vi "Process.vi"(8 "error in":errorcluster, 11 "Transport":refnum<class "Transport.lvclass">) -> (0 "error out":errorcluster, 3 "Transport out":refnum<class "Transport.lvclass">)   [LabVIEW 2016, in "Transport.lvclass"]
doc: "---------------------------------------------------------------\nJKI State Machine Objects™\nhttp://jki.net/state-machine-objects/\nCopyright (C) 2005-2015, JKI <info@jki.net>\nALL RIGHTS RESERVED"
uses:
  Transport.lvclass
  <vilib>/JKI/JKI SMO/SMO/SMO.lvclass
  <vilib>/JKI/JKI SMO/SMO/Typedefs/Parent Call--Enum.ctl
  Control Experiment/Control Experiment.lvclass
  <userlib>/LevyLab/Lockin-Multichannel/Instrument.Lockin/Instrument.Lockin.lvclass
  <userlib>/LevyLab/Levylab Instruments/Instrument Types/Cryostat/Typedefs/Magnet Axis--Enum.ctl
  <userlib>/LevyLab/Levylab Instruments/Instrument Types/Cryostat/Instrument.Cryostat.lvclass
  <userlib>/LevyLab/Levylab Instruments/Instrument Types/Cryostat/Typedefs/Magnet Mode--Enum.ctl
  <userlib>/LevyLab/Levylab Instruments/Instrument Types/Strain/Instrument.Strain.lvclass
  <userlib>/LevyLab/Levylab Instruments/Instrument Types/Optical Delay Line/Instrument.OpticalDelayLine.lvclass
  <userlib>/LevyLab/Levylab Instruments/Instrument Types/CBridge/Instrument.CBridge.lvclass
  C:/Program Files (x86)/National Instruments/LabVIEW 2016/vi.lib/JKI/JKI SMO/SMO/SMO.lvclass
panel:
  # "For instructions on how to use the JKI State Machine Objects, examples and video tutorials, visit:\nhttp://jki.net/state-machine-objects/\n\nJKI State Machine Objects™\nhttp://jki.net/state-machine-objects/\nCopyright (C) 2005-2015, JKI <info@jki.net>\nALL RIGHTS RESERVED"
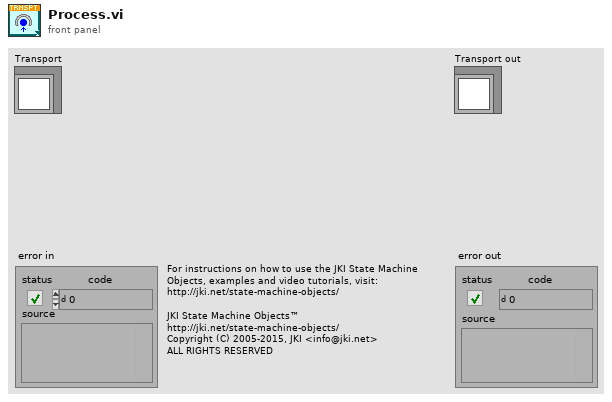
[diagram p1: front panel]
types:
  T1 = typedef "SMO.lvclass/Parent Call--Enum.ctl" = enum16{"Allows parent to run", "Does not request parent to run"}
  T2 = enum32{"invalid app kind", "Development System", "Run Time System", "Student Edition", "Embedded LabVIEW", "Evaluation", "Custom"}
  T3 = enum32{"Invalid", "Standard", "Closed", "Hidden", "Minimized", "Maximized"}
  T4 = enum32{"Bad", "Idle", "Run top level", "Running"}
  T5 = typedef "Instrument.Cryostat.lvclass/Magnet Mode--Enum.ctl" = enum16{"Persistent", "Driven"}
  T6 = typedef "Instrument.Cryostat.lvclass/Magnet Axis--Enum.ctl" = enum16{"Z", "X", "Y"}
  T7 = typedef "Control Experiment.lvclass/Instruments--cluster.ctl" = cluster{"Lockin":refnum<class "Instrument.Lockin.lvclass">, "Temperature":refnum<class "Instrument.Cryostat.lvclass">, "Magnet":refnum<class "Instrument.Cryostat.lvclass">, "Rotator":refnum<class "Instrument.Cryostat.lvclass">, "Level":refnum<class "Instrument.Cryostat.lvclass">, "C Bridge":refnum<class "Instrument.CBridge.lvclass">, "Optical Delay Line":refnum<class "Instrument.OpticalDelayLine.lvclass">, "Strain Cell":refnum<class "Instrument.Strain.lvclass">, "VNA":refnum<class "Instrument.VNA.lvclass">, "Voltage Source":refnum<class "Instrument.VSource.lvclass">, "KH7008":refnum<class "Instrument.KH7008.lvclass">[]}
  T8 = cluster{"Core":cluster{"Current VI Reference":refnum<vi>, "Close Panel on Exit?":bool, "error":errorcluster}, "Self Reference":refnum<class "Transport.lvclass">, "Control Experiment":refnum<class "Control Experiment.lvclass">, "Instruments":T7, "value":variant, "wait":bool}
  T9 = cluster{"Current VI Reference":refnum<vi>, "Close Panel on Exit?":bool, "error":errorcluster}
  T10 = typedef "SMO.lvclass/Protected Events.ctl" = cluster{"StopProcesses":refnum<user-event>, "AbortProcesses":refnum<user-event>, "Config Changed":refnum<user-event>, "Dependency":refnum<user-event>}
  T11 = typedef "Transport.lvclass/PrivateEvents--Cluster.ctl" = cluster{"Configure":refnum<user-event>}
  T12 = typedef "Lockin.DAQ.lvclass/State-enum.ctl" = enum16{"idle", "created", "started", "stopped", "sweeping"}
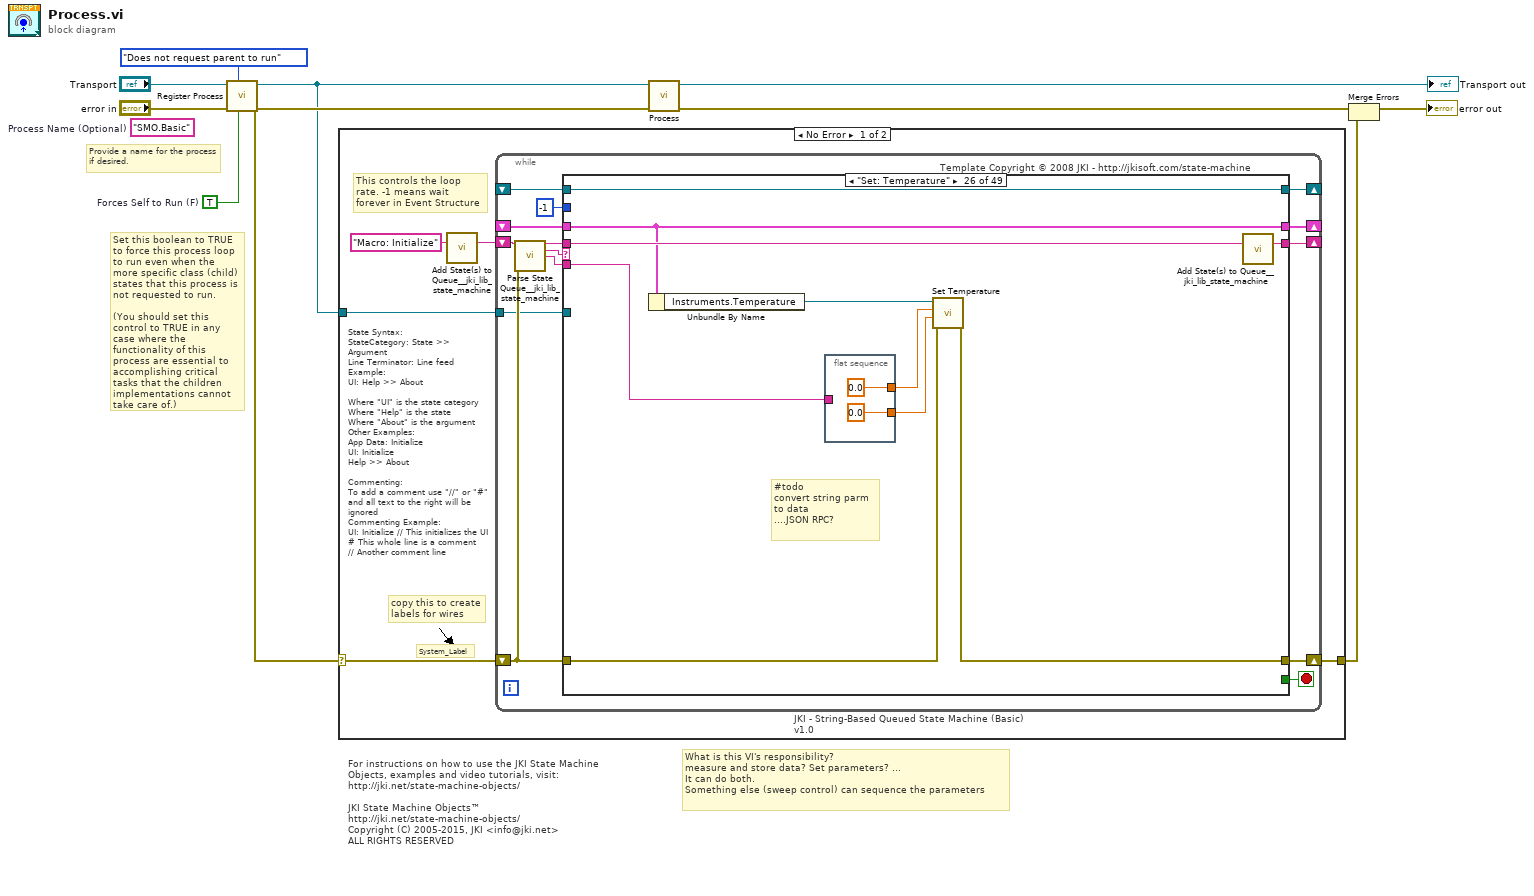
[diagram p0: block diagram]
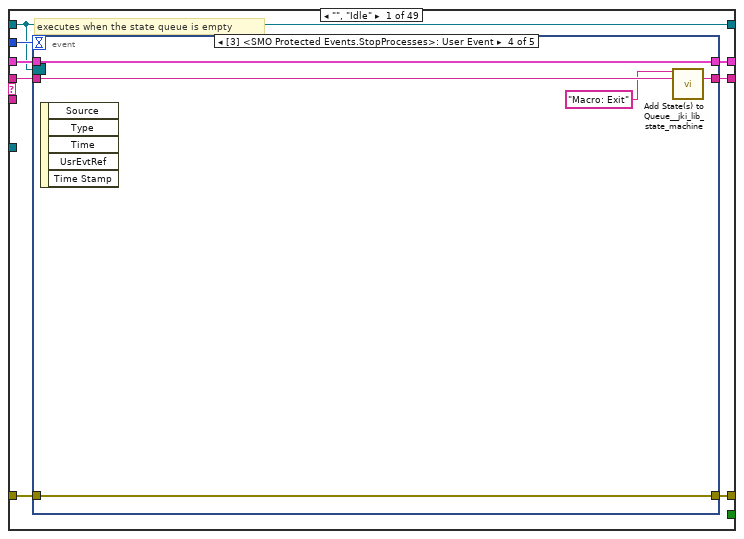
[diagram p2: hidden frame]
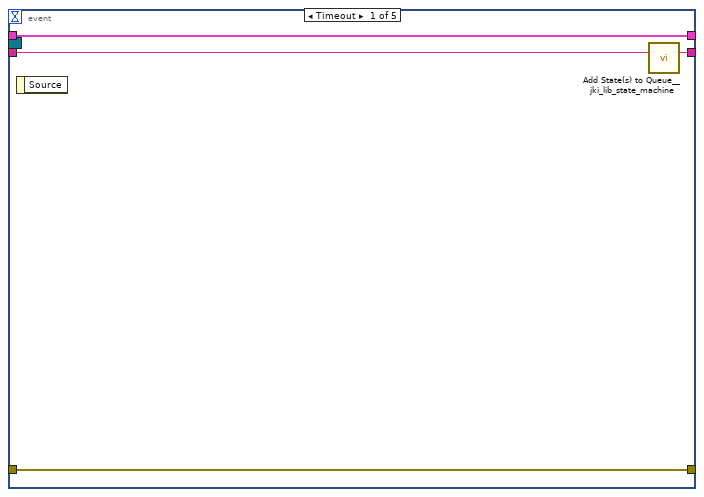
[diagram p3: hidden frame]
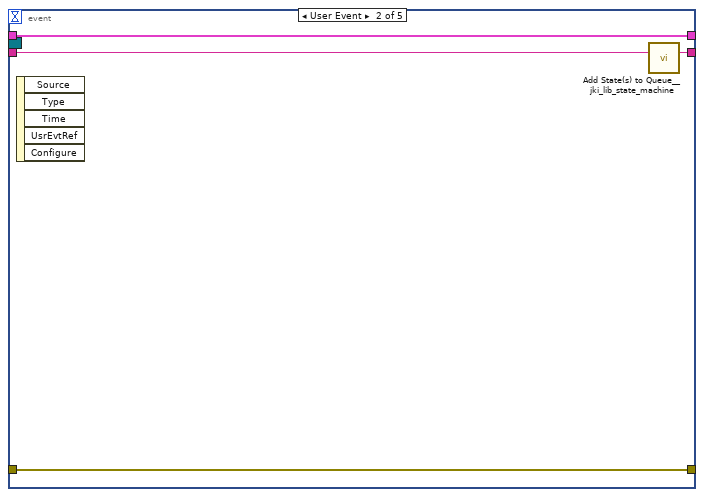
[diagram p4: hidden frame]
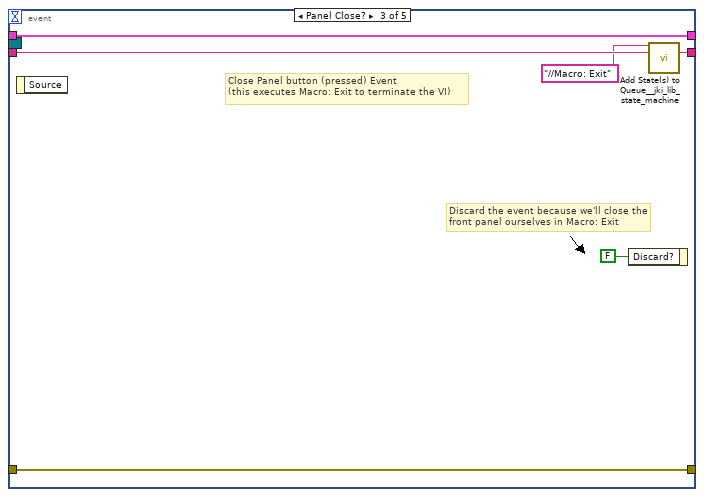
[diagram p5: hidden frame]
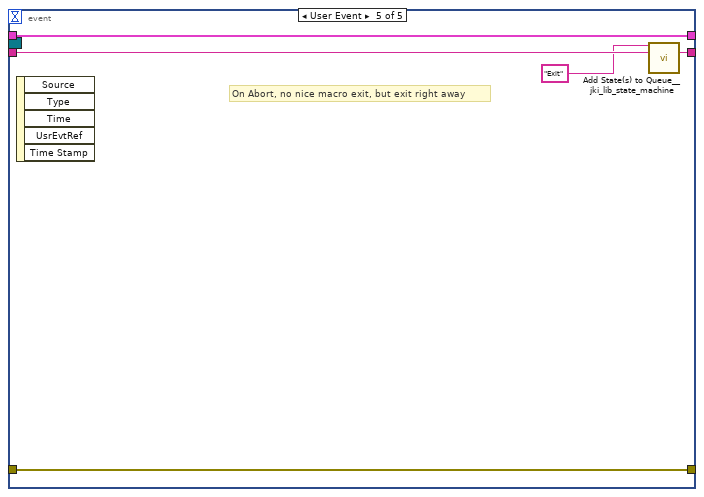
[diagram p6: hidden frame]
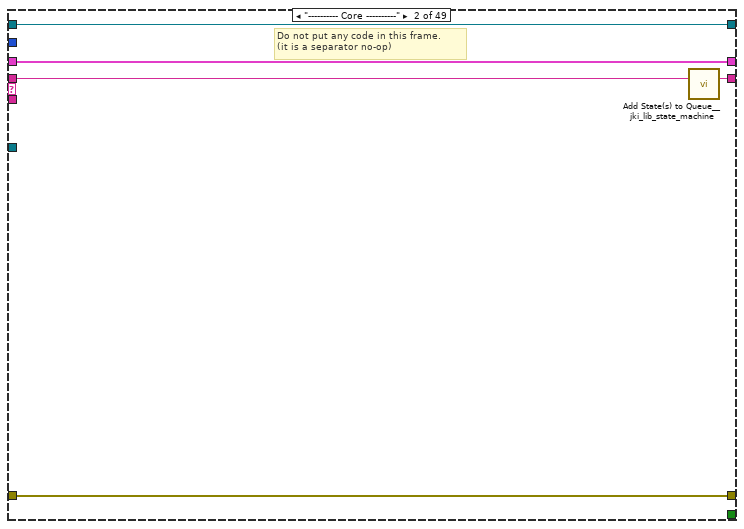
[diagram p7: hidden frame]
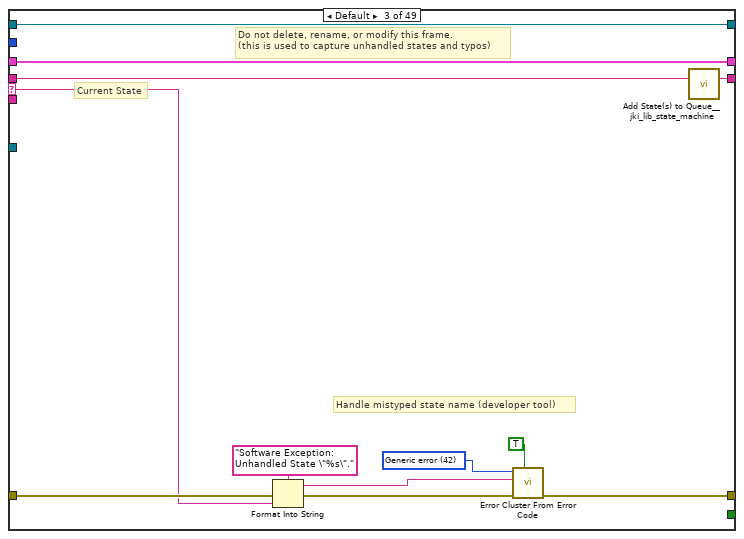
[diagram p8: hidden frame]
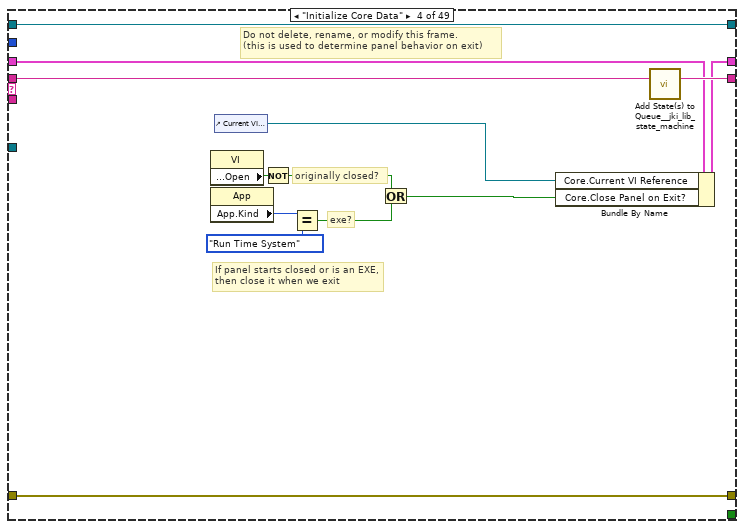
[diagram p9: hidden frame]
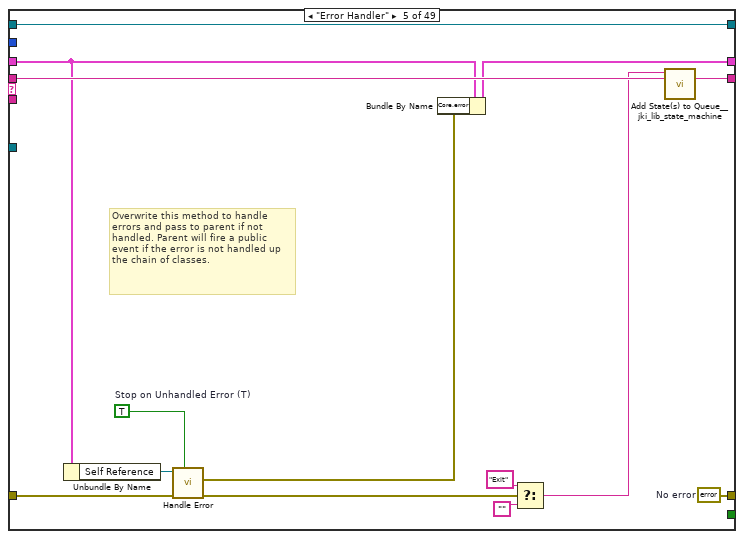
[diagram p10: hidden frame]
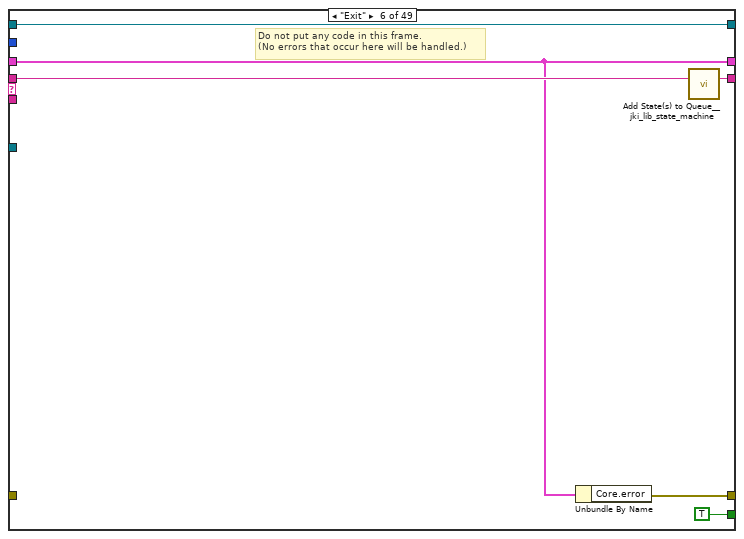
[diagram p11: hidden frame]
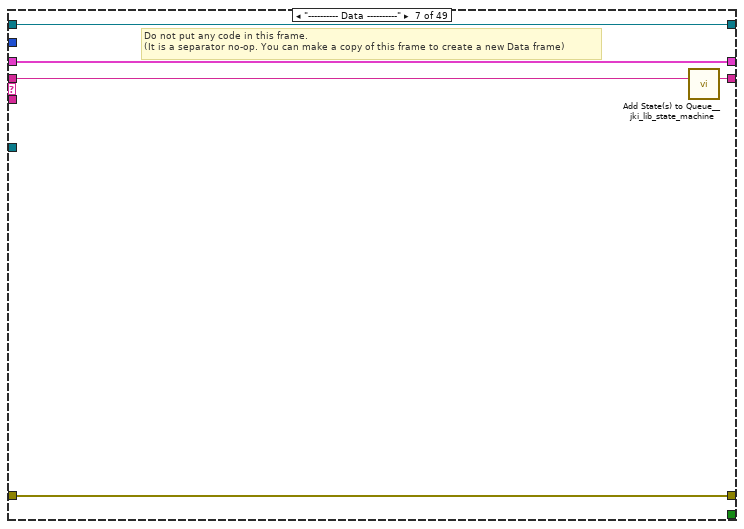
[diagram p12: hidden frame]
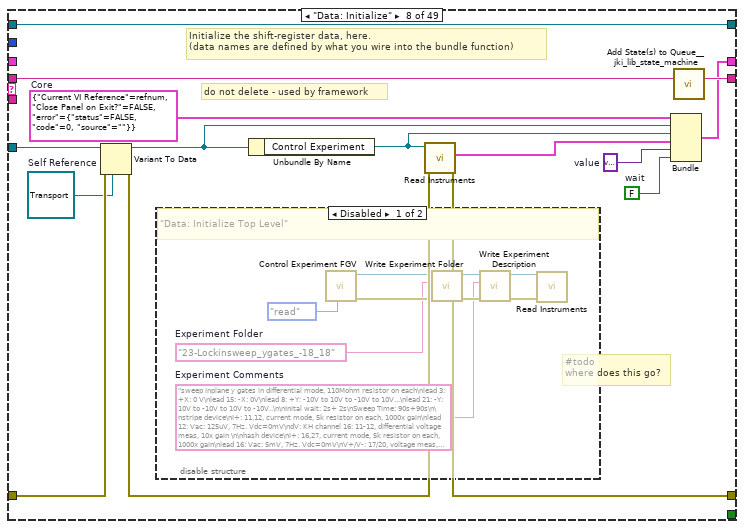
[diagram p13: hidden frame]
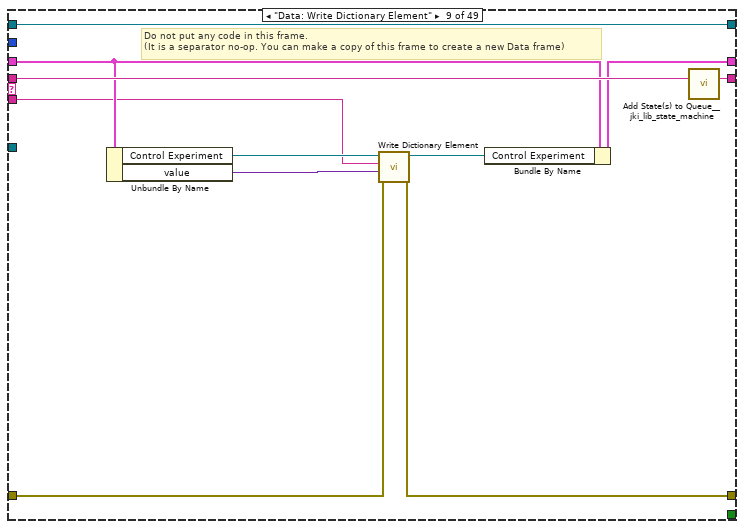
[diagram p15: hidden frame]
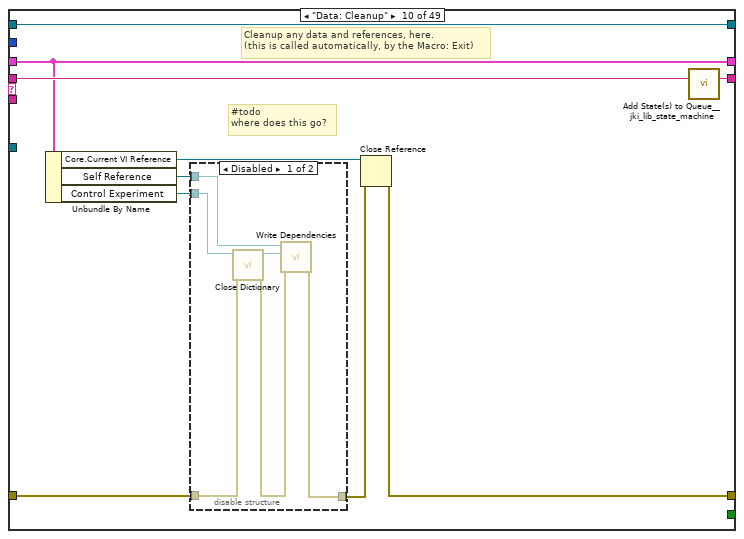
[diagram p16: hidden frame]
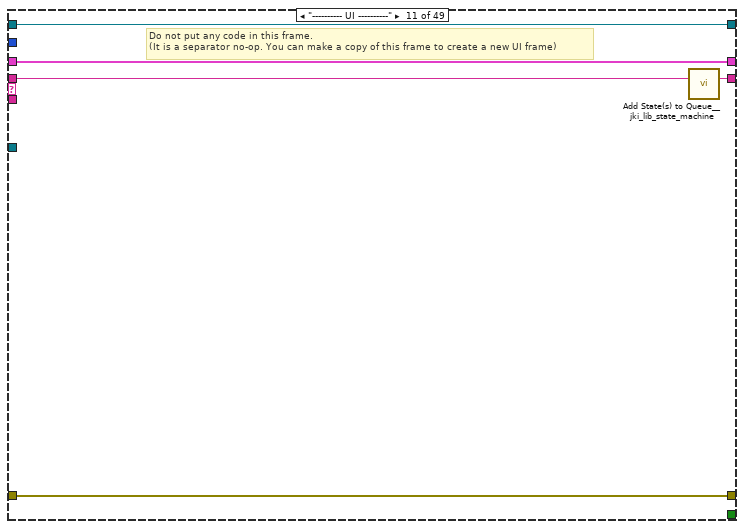
[diagram p18: hidden frame]
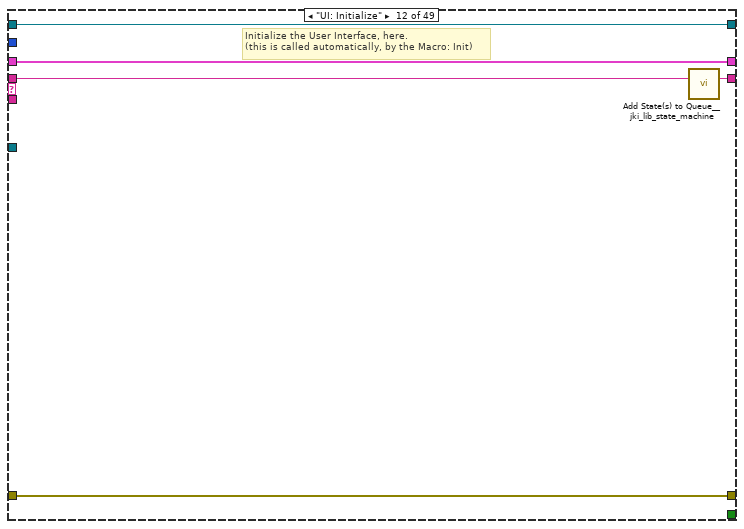
[diagram p19: hidden frame]
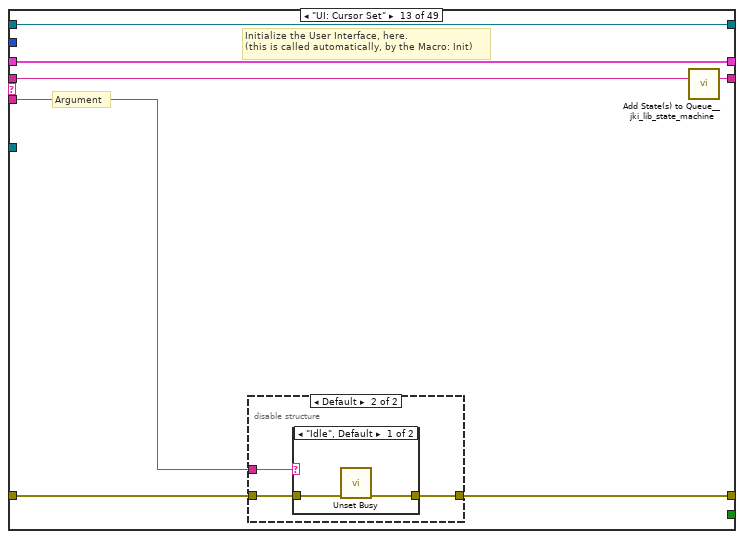
[diagram p20: hidden frame]
diagram:
  w1 = TRUE  # Forces Self to Run (F)
  (unwired) "SMO.Basic"  # Process Name (Optional)
  # "What is this VI's responsibility?\nmeasure and store data? Set parameters? ...\nIt can do both.\nSomething else (sweep control) can sequence the parameters"
  # "Provide a name for the process\nif desired."
  # "Set this boolean to TRUE to force this process loop to run even when the more specific class (child) states that this process is not requested to run.\n\n(You should set this control to TRUE in any case where the functionality of this process are essential to accomplishing critical tasks that the children implementations cannot take care of.)"
  # "For instructions on how to use the JKI State Machine Objects, examples and video tutorials, visit:\nhttp://jki.net/state-machine-objects/\n\nJKI State Machine Objects™\nhttp://jki.net/state-machine-objects/\nCopyright (C) 2005-2015, JKI <info@jki.net>\nALL RIGHTS RESERVED"
  n1 = call <vilib>:"Register Process.vi"("Forces Self to Run (F)"=w1, "Parent Call"=Parent_Call--Enum."Does not request parent to run", "error in (no error)"="error in", "SMO"="Transport") -> ("error out"=w7:errorcluster, "SMO out"=w6:refnum<class "Transport.lvclass">)  [unwired: 6 in]
  n2 = case shown="No Error" w7 {
    selector: w7 -> [w12 w561]
    tunnel: w6 -> [w13 _]
    tunnel: [w11 w561] -> w3
    frame No Error {
      # "State Syntax:\nStateCategory: State >> Argument\nLine Terminator: Line feed\nExample:\nUI: Help >> About\n\nWhere \"UI\" is the state category\nWhere \"Help\" is the state\nWhere \"About\" is the argument\nOther Examples:\nApp Data: Initialize\nUI: Initialize\nHelp >> About\n\nCommenting:\nTo add a comment use \"//\" or \"#\" and all text to the right will be ignored\nCommenting Example:\nUI: Initialize // This initializes the UI\n# This whole line is a comment\n// Another comment line"
      # "copy this to create labels for wires"
      # "This controls the loop rate. -1 means wait forever in Event Structure"
      # "System_Label"
      n3 = call <vilib>:"Add State(s) to Queue__jki_lib_state_machine.vi"("State(s) in (\"\")"="Macro: Initialize") -> ("States Out"=w15:string)  [unwired: 14 in]
      n4 = while "JKI - String-Based Queued State Machine (Basic) v1.0" {
        shift-right: [w22] -> _
        shift-left: _ -> [w21]
        shift-right: [w25] -> w11
        shift-left: w12 -> [w19]
        shift-right: [w24] -> _
        shift-left: w15 -> [w26]
        tunnel: w13 -> [w18]
        shift-right: [w17] -> _
        shift-left: _ -> [w16]
        stop <- w23 stop-if-true
        # "Template Copyright © 2008 JKI - http://jkisoft.com/state-machine"
        n5 = call <vilib>:"Parse State Queue__jki_lib_state_machine.vi"("State Queue"=w26, "Error In (no error)"=w19) -> ("Remaining States"=w28:string, "Current State"=w29:string, "Arguments"=w27:string)  [unwired: 11 in]
        n6 = case shown="\"Set: Temperature\"" w29 {
          selector: w29 -> [_ _ w68 _ _ _ _ _ _ _ _ _ _ _ _ _ _ _ _ _ _ _ _ _ w313 _ _ _ _ _ _ _ _ _ _ _ _ _ _ _ _ _ _ _ _ _ _ _ _]
          tunnel: w28 -> [w37 w66 w72 w91 w105 w111 w116 w131 w151 w161 w173 w178 w185 w201 w233 w247 w252 w266 w271 w282 w287 w299 w305 w310 w325 w335 w349 w363 w375 w387 w399 w411 w423 w435 w442 w449 w458 w467 w475 w480 w488 w497 w506 w515 w524 w533 w542 w551 w560]
          tunnel: w27 -> [_ _ _ _ _ _ _ _ w141 _ _ _ w179 w195 _ _ _ _ _ _ _ _ _ _ w314 w326 w344 w358 w370 w382 w394 w406 w418 w430 _ _ _ _ _ _ _ _ _ _ _ _ _ _ _]
          tunnel: w21 -> [w35 w63 w70 w82 w99 w107 w113 _ w146 w152 w170 w176 w183 w197 w230 w243 w249 w257 w268 w279 w284 w297 w303 w307 w321 w331 w345 w359 w371 w383 w395 w407 w419 w431 w439 w446 w455 w464 w472 w478 w485 w491 w500 w509 w518 w527 w536 w545 w554]
          tunnel: [w34 w64 w74 w88 w100 w106 w114 w119 w143 w158 w171 w175 w180 w198 w231 w245 w250 w264 w269 w273 w285 w293 w301 w308 w323 w332 w346 w360 w372 w384 w396 w408 w420 w432 w440 w443 w450 w459 w469 w476 w482 w493 w502 w511 w520 w529 w538 w547 w556] -> w25
          tunnel: w19 -> [w33 w64 w73 w88 w101 _ w114 w128 w144 w154 w171 w175 w181 w199 w231 w245 w250 w264 w269 w274 w285 w294 w301 w308 w323 w327 w338 w354 w366 w378 w390 w402 w414 w426 w440 w444 w453 w462 w470 w476 w482 w489 w498 w507 w516 w525 w534 w543 w552]
          tunnel: [w36 w65 w71 w90 w104 w110 w115 w130 w150 w160 w172 w177 w184 w200 w232 w246 w251 w265 w270 w281 w286 w298 w304 w309 w324 w334 w348 w362 w374 w386 w398 w410 w422 w434 w441 w448 w457 w466 w474 w479 w487 w496 w505 w514 w523 w532 w541 w550 w559] -> w24
          tunnel: [_ _ _ _ _ TRUE _ _ _ _ _ _ _ _ _ _ _ _ _ _ _ _ _ _ _ _ _ _ _ _ _ _ _ _ _ _ _ _ _ _ _ _ _ _ _ _ _ _ _] -> w23
          tunnel: [w32 w63 w70 w89 w98 w107 w113 w129 w145 w152 w170 w176 w183 w197 w230 w243 w249 w257 w268 w279 w284 w297 w303 w307 w320 w331 w345 w359 w371 w383 w395 w407 w419 w431 w439 w446 w455 w464 w472 w478 w484 w494 w503 w512 w521 w530 w539 w548 w557] -> w22
          tunnel: -1 ("Timeout") -> [w31 _ _ _ _ _ _ _ _ _ _ _ _ _ _ _ _ _ _ _ _ _ _ _ _ _ _ _ _ _ _ _ _ _ _ _ _ _ _ _ _ _ _ _ _ _ _ _ _]
          tunnel: w18 -> [_ _ _ _ _ _ _ w127 _ _ _ _ _ _ _ _ _ _ _ _ _ _ _ _ _ _ _ _ _ _ _ _ _ _ _ _ _ _ _ _ _ _ _ _ _ _ _ _ _]
          tunnel: [w30 w62 w67 w79 w103 w108 w112 w126 w149 w157 w169 w174 w182 w194 w229 w244 w248 w258 w267 w280 w283 w296 w302 w306 w322 w333 w347 w361 w373 w385 w397 w409 w421 w433 w438 w447 w456 w465 w473 w477 w486 w495 w504 w513 w522 w531 w540 w549 w558] -> w17
          tunnel: w16 -> [w30 w62 w67 w79 w103 w108 w112 w126 w149 w157 w169 w174 w182 w194 w229 w244 w248 w258 w267 w280 w283 _ w302 w306 w322 w333 w347 w361 w373 w385 w397 w409 w421 w433 w438 w447 w456 w465 w473 w477 w486 w495 w504 w513 w522 w531 w540 w549 w558]
          frame "", "Idle" {
            # "executes when the state queue is empty"
            n7 = event shown="[3] <SMO Protected Events.StopProcesses>: User Event" {
              selector: w30 -> [_ _ _ _ _]
              dyn-events: _ -> [_ _ _ _ _]
              timeout: w31 -> [_ _ _ _ _]
              tunnel: w37 -> [w41 w45 w51 w56 w61]
              tunnel: [w40 w44 w50 w55 w60] -> w36
              tunnel: w35 -> [w39 w43 w48 w53 w58]
              tunnel: [w38 w42 w49 w54 w59] -> w34
              tunnel: w33 -> [w38 w42 w49 w54 w59]
              tunnel: [w39 w43 w48 w53 w58] -> w32
              event Timeout {
                n8 = event-data() -> ()  [unwired: 1 in, 1 out]
                n9 = call <vilib>:"Add State(s) to Queue__jki_lib_state_machine.vi"("State(s) in (\"\")"=w41) -> ("States Out"=w40:string)  [unwired: 14 in]
              }
              event User Event {
                n10 = event-data() -> ()  [unwired: 1 in, 5 out]
                n11 = call <vilib>:"Add State(s) to Queue__jki_lib_state_machine.vi"("State(s) in (\"\")"=w45) -> ("States Out"=w44:string)  [unwired: 14 in]
              }
              event Panel Close? {
                # "Discard the event because we'll close the front panel ourselves in Macro: Exit"
                # "Close Panel button (pressed) Event\n(this executes Macro: Exit to terminate the VI)"
                n12 = event-data() -> ()  [unwired: 1 in, 1 out]
                n13 = event-data("Discard?"=FALSE) -> ()  [unwired: 1 in, 1 out]
                n14 = call <vilib>:"Add State(s) to Queue__jki_lib_state_machine.vi"("State(s) in Front (\"\")"="//Macro: Exit", "State(s) in (\"\")"=w51) -> ("States Out"=w50:string)  [unwired: 13 in]
              }
              event User Event {
                n15 = event-data() -> ()  [unwired: 1 in, 5 out]
                n16 = call <vilib>:"Add State(s) to Queue__jki_lib_state_machine.vi"("State(s) in Front (\"\")"="Macro: Exit", "State(s) in (\"\")"=w56) -> ("States Out"=w55:string)  [unwired: 13 in]
              }
              event User Event {
                # "On Abort, no nice macro exit, but exit right away"
                n17 = event-data() -> ()  [unwired: 1 in, 5 out]
                n18 = call <vilib>:"Add State(s) to Queue__jki_lib_state_machine.vi"("State(s) in Front (\"\")"="Exit", "State(s) in (\"\")"=w61) -> ("States Out"=w60:string)  [unwired: 13 in]
              }
            }
          }
          frame "---------- Core ----------" {
            # "Do not put any code in this frame.\n(it is a separator no-op)"
            n19 = call <vilib>:"Add State(s) to Queue__jki_lib_state_machine.vi"("State(s) in (\"\")"=w66) -> ("States Out"=w65:string)  [unwired: 14 in]
          }
          frame Default {
            w77 = 42 items=["No error", "Argument error", "Memory is full", "Out of zone", "End of file", "File already open", "Generic file I/O error", "File not found", "File permission error", "Disk is full", "Duplicate path", "Too many files open", "System feature not enabled", "Resource file not found", "Cannot add resource", "Resource not found", "Image not found", "Image memory error", "Pen does not exist", "Config type invalid", "Config token not found", "Config parse error", "Config memory error", "Bad external code format", "Bad external code offset", "External code not present", "Null window", "Destroy window error", "Null menu", "Print aborted", "Bad print record", "Print driver error", "Windows error during printing", "Memory error during printing", "Print dialog error", "Generic print error", "Invalid device refnum", "Device not found", "Device parameter error", "Device unit error", "Cannot open device", "Device call aborted", "Generic error", "Cancelled by user", "Object ID too low", "Object ID too high", "Object not in heap", "Unknown heap", "Unknown object (invalid DefProc)", "Unknown object (DefProc not in table)", "Message out of range", "Invalid (null) method", "Unknown message", "Manager call not supported", "Bad address", "Network operation in progress", "Network operation timed out", "Connection is busy", "Network attribute not supported", "Network error", "Address in use", "System out of memory", "Connection aborted", "Connection refused", "Not connected", "Already connected", "Connection closed", "Initialization error (interapplication manager)", "Bad occurrence", "Wait on unbound occurrence handler", "Occurrence queue overflow", "Datalog type conflict", "Unused", "Unrecognized type (interapplication manager)", "Memory corrupt", "Failed to make temporary DLL", "Old CIN version", "Drag socket not found", "Failed to load drop-object", "Failed to register OLE object", "Failed to release OLE object", "Format specifier type mismatch", "Unknown format specifier", "Too few format specifiers", "Too many format specifiers", "Scan failed", "Newer CIN version", "Error converting to variant", "Runtime menu error", "Password tampered", "Variant attribute not found", "Incompatible variant data type", "Event data is not available", "Event Store is not present", "Occurrence is not found", "Event Queue is not created", "Event info is not available", "Refnum passed is NULL", "Error retrieving Class GUID", "Error retrieving CoClass GUID", "Error retrieving TypeLib GUID.", "Bad built application magic bytes.", "Specific driver is different from the specific driver associated with the Logical Name.", "There is no session opened to the class driver.", "Max Error", "MAX - Error with config objects", "MAX - Error loading configuration", "MAX - Group not supported"]
            # "Current State"
            # "Do not delete, rename, or modify this frame.\n(this is used to capture unhandled states and typos)"
            # "Handle mistyped state name (developer tool)"
            n20 = Format Into String(format string="Software Exception: Unhandled State \"%s\"." ("message"), error in=w73, w68) -> (resulting string=w76:string, error out=w75:errorcluster)  [unwired: 1 in]
            n21 = call <vilib>:"Error Cluster From Error Code.vi"("show call chain? (False)"=TRUE, "error in (no error)"=w75, "error message (\"\")"=w76, "error code (0)"=w77) -> ("error out"=w74:errorcluster)  [unwired: 5 in]
            n22 = call <vilib>:"Add State(s) to Queue__jki_lib_state_machine.vi"("State(s) in (\"\")"=w72) -> ("States Out"=w71:string)  [unwired: 14 in]
          }
          frame "Initialize Core Data" {
            # "Do not delete, rename, or modify this frame.\n(this is used to determine panel behavior on exit)"
            # "originally closed?"
            # "exe?"
            # "If panel starts closed or is an EXE, then close it when we exit"
            n23 = property class="VI"() -> ("Front Panel.Open"=w87:bool)  [unwired: 2 in, 2 out]
            n24 = property class="App"() -> ("App.Kind"=w86:T2)  [unwired: 2 in, 2 out]
            n25 = control-ref of="Current VI Reference"() -> (w80:refnum<vi>)
            n26 = Not(x=w87) -> (.not. x?=w84:bool)
            n27 = Equal?(x=w86, y=T2."Run Time System" ("Application:Kind")) -> (x = y?=w83:bool)
            n28 = Or(x=w84, y=w83) -> (x .or. y?=w81:bool)
            n29 = Bundle By Name(cluster=w82, "Core.Current VI Reference"=w80, "Core.Close Panel on Exit?"=w81) -> (w89:T8)
            n30 = call <vilib>:"Add State(s) to Queue__jki_lib_state_machine.vi"("State(s) in (\"\")"=w91) -> ("States Out"=w90:string)  [unwired: 14 in]
          }
          frame "Error Handler" {
            w92 = TRUE  # Stop on Unhandled Error (T)
            w100 = errorcluster {"status"=FALSE, "code"=0, "source"=""}  # No error
            # "Overwrite this method to handle errors and pass to parent if not handled. Parent will fire a public event if the error is not handled up the chain of classes."
            n31 = Unbundle By Name(w99) -> ("Self Reference"=w102:refnum<class "Transport.lvclass">)
            n32 = call-dynamic "Handle Error.vi"("Stop on Unhandled Error (T)"=w92, "error in"=w101, "SMO"=w102) -> ("handling error"=w93:errorcluster, "Unhandled error"=w96:errorcluster)  [unwired: 6 in, 1 out]
            n33 = Bundle By Name(cluster=w99, "Core.error"=w96) -> (w98:T8)
            n34 = Select(t="Exit", s=w93, f="") -> (s? t:f=w97:string)
            n35 = call <vilib>:"Add State(s) to Queue__jki_lib_state_machine.vi"("State(s) in Front (\"\")"=w97, "State(s) in (\"\")"=w105) -> ("States Out"=w104:string)  [unwired: 13 in]
          }
          frame "Exit" {
            # "Do not put any code in this frame.\n(No errors that occur here will be handled.)"
            n36 = Unbundle By Name(w107) -> ("Core.error"=w106:errorcluster)
            n37 = call <vilib>:"Add State(s) to Queue__jki_lib_state_machine.vi"("State(s) in (\"\")"=w111) -> ("States Out"=w110:string)  [unwired: 14 in]
          }
          frame "---------- Data ----------" {
            # "Do not put any code in this frame.\n(It is a separator no-op. You can make a copy of this frame to create a new Data frame)"
            n38 = call <vilib>:"Add State(s) to Queue__jki_lib_state_machine.vi"("State(s) in (\"\")"=w116) -> ("States Out"=w115:string)  [unwired: 14 in]
          }
          frame "Data: Initialize" {
            w118 = FALSE  # wait
            w123 = variant  # value
            w124 = refnum<class "Transport.lvclass"> refnum  # Self Reference
            w125 = T9 {"Current VI Reference"=refnum, "Close Panel on Exit?"=FALSE, "error"={"status"=FALSE, "code"=0, "source"=""}}  # Core
            # "#todo\nwhere does this go?"
            # "do not delete - used by framework"
            # "Initialize the shift-register data, here.\n(data names are defined by what you wire into the bundle function)"
            n39 = Variant To Data(error in=w128, type=w124, Variant=w127) -> (data=w117:refnum<class "Transport.lvclass">, error out=w120:errorcluster)
            n40 = disable-structure shown="Disabled" {
              frame Disabled {
                w134 = "sweep inplane y gates in differential mode, 110Mohm resistor on each\nlead 3: +X: 0 V\nlead 15: -X: 0V\nlead 8: +Y: -10V to 10V to -10V to 10V...\nlead 21: -Y: 10V to -10V to 10V to -10V..\n\nInital wait: 2s+ 2s\nSweep Time: 90s+90s\n\nstripe device\nI+: 11,12, current mode, 5k resistor on each, 1000x gain\nlead 12: Vac: 125uV, 7Hz. Vdc=0mV\ndV: KH channel 16: 11-12, differential voltage meas, 10x gain \n\nhash device\nI+: 16,27, current mode, 5k resistor on each, 1000x gain\nlead 16: Vac: 5mV, 7Hz. Vdc=0mV\nV+/V-: 17/20, voltage meas, 10x gain \nKH 5: 17-20, volt. meas., 10x gain\n\n\nlead 26: Vbg: 0V, 1Gohm resistor\nB: -18T to 18T @0.033T/min\n"  # Experiment Comments
                w135 = "23-Lockinsweep_ygates_-18_18"  # Experiment Folder
                # "\"Data: Initialize Top Level\""
                n41 = call "Control Experiment FGV.vi"("Function"=enum16{"read", "write"}."read") -> ("error out"=w139:errorcluster, "Control Experiment out"=w140:refnum<class "Control Experiment.lvclass">)  [unwired: 9 in]
                n42 = call "Write Experiment Folder.vi"("error in (no error)"=w139, "Experiment Folder"=w135, "Control Experiment"=w140) -> ("error out"=w137:errorcluster, "Control Experiment out"=w138:refnum<class "Control Experiment.lvclass">)  [unwired: 7 in]
                n43 = call "Write Experiment Description.vi"("error in (no error)"=w137, "Experiment Description"=w134, "Control Experiment"=w138) -> ("error out"=w132:errorcluster, "Control Experiment out"=w133:refnum<class "Control Experiment.lvclass">)  [unwired: 7 in]
                n44 = call "Read Instruments.vi"("error in (no error)"=w132, "Control Experiment"=w133) -> ()  [unwired: 7 in, 3 out]
              }
              frame Enabled {
              }
            }
            n45 = Unbundle By Name(w117) -> ("Control Experiment"=w122:refnum<class "Control Experiment.lvclass">)
            n46 = call "Read Instruments.vi"("error in (no error)"=w120, "Control Experiment"=w122) -> ("error out"=w119:errorcluster, "Instruments"=w121:T7)  [unwired: 7 in, 1 out]
            n47 = Bundle("Core"=w125, "Self Reference"=w117, "Control Experiment"=w122, "Instruments"=w121, "value"=w123, "wait"=w118) -> (w129:T8)  [unwired: 1 in]
            n48 = call <vilib>:"Add State(s) to Queue__jki_lib_state_machine.vi"("State(s) in (\"\")"=w131) -> ("States Out"=w130:string)  [unwired: 14 in]
          }
          frame "Data: Write Dictionary Element" {
            # "Do not put any code in this frame.\n(It is a separator no-op. You can make a copy of this frame to create a new Data frame)"
            n49 = Unbundle By Name(w146) -> ("Control Experiment"=w148:refnum<class "Control Experiment.lvclass">, "value"=w142:variant)
            n50 = call "Write Dictionary Element.vi"("error in (no error)"=w144, "value"=w142, "key"=w141, "Control Experiment"=w148) -> ("error out"=w143:errorcluster, "Control Experiment out"=w147:refnum<class "Control Experiment.lvclass">)  [unwired: 6 in]
            n51 = Bundle By Name(cluster=w146, "Control Experiment"=w147) -> (w145:T8)
            n52 = call <vilib>:"Add State(s) to Queue__jki_lib_state_machine.vi"("State(s) in (\"\")"=w151) -> ("States Out"=w150:string)  [unwired: 14 in]
          }
          frame "Data: Cleanup" {
            # "#todo\nwhere does this go?"
            # "Cleanup any data and references, here.\n(this is called automatically, by the Macro: Exit)"
            n53 = Unbundle By Name(w152) -> ("Core.Current VI Reference"=w159:refnum<vi>, "Self Reference"=w156:refnum<class "Transport.lvclass">, "Control Experiment"=w155:refnum<class "Control Experiment.lvclass">)
            n54 = disable-structure shown="Disabled" {
              disable-tunnel: w156 -> [w162 _]
              disable-tunnel: w155 -> [w163 _]
              disable-tunnel: w154 -> [w166 w168]
              disable-tunnel: [w164 w168] -> w153
              frame Disabled {
                n55 = call "Close Dictionary.vi"("error in (no error)"=w166, "Control Experiment"=w163) -> ("error out"=w165:errorcluster, "Control Experiment out"=w167:refnum<class "Control Experiment.lvclass">)  [unwired: 8 in]
                n56 = call "Write Dependencies.vi"("error in (no error)"=w165, "Control Experiment"=w167, "Transport in"=w162) -> ("error out"=w164:errorcluster)  [unwired: 7 in, 1 out]
              }
              frame Enabled {
              }
            }
            n57 = Close Reference(reference=w159, error in (no error)=w153) -> (error out=w158:errorcluster)
            n58 = call <vilib>:"Add State(s) to Queue__jki_lib_state_machine.vi"("State(s) in (\"\")"=w161) -> ("States Out"=w160:string)  [unwired: 14 in]
          }
          frame "---------- UI ----------" {
            # "Do not put any code in this frame.\n(It is a separator no-op. You can make a copy of this frame to create a new UI frame)"
            n59 = call <vilib>:"Add State(s) to Queue__jki_lib_state_machine.vi"("State(s) in (\"\")"=w173) -> ("States Out"=w172:string)  [unwired: 14 in]
          }
          frame "UI: Initialize" {
            # "Initialize the User Interface, here.\n(this is called automatically, by the Macro: Init)"
            n60 = call <vilib>:"Add State(s) to Queue__jki_lib_state_machine.vi"("State(s) in (\"\")"=w178) -> ("States Out"=w177:string)  [unwired: 14 in]
          }
          frame "UI: Cursor Set" {
            # "Argument"
            # "Initialize the User Interface, here.\n(this is called automatically, by the Macro: Init)"
            n61 = disable-structure shown="Default" {
              disable-tunnel: w181 -> [w186 w189]
              disable-tunnel: [w186 w188] -> w180
              disable-tunnel: w179 -> [_ w187]
              frame condition #0 {
              }
              frame condition #1 (active) {
                n62 = case shown="\"Idle\", Default" w187 {
                  tunnel: w189 -> [w191 w193]
                  tunnel: [w190 w192] -> w188
                  frame "Idle", Default {
                    n63 = call <vilib>:"Unset Busy.vi"("error in (no error)"=w191) -> ("error out"=w190:errorcluster)  [unwired: 10 in]
                  }
                  frame "Busy" {
                    n64 = call <vilib>:"Set Busy.vi"("error in (no error)"=w193) -> ("error out"=w192:errorcluster)  [unwired: 9 in, 1 out]
                  }
                }
              }
            }
            n65 = call <vilib>:"Add State(s) to Queue__jki_lib_state_machine.vi"("State(s) in (\"\")"=w185) -> ("States Out"=w184:string)  [unwired: 14 in]
          }
          frame "UI: Front Panel State" {
            # "Argument"
            # "Set Front Panel Open or Closed\n(Usage: \"UI: Front Panel State >> Open|Close\")"
            n66 = Unbundle By Name(w197) -> ("Core.Current VI Reference"=w196:refnum<vi>)
            n67 = disable-structure shown="Default" {
              disable-tunnel: w199 -> [w205 w228]
              disable-tunnel: [w204 w228] -> w198
              disable-tunnel: w196 -> [w203 _]
              disable-tunnel: w195 -> [w202 _]
              frame condition #0 (active) {
                n68 = case shown="\"Close\"" w202 {
                  tunnel: w205 -> [w209 w222]
                  tunnel: [w211 w223] -> w204
                  tunnel: w203 -> [w210 w220]
                  frame "Open", Default {
                    n69 = property class="VI"(reference=w210, error in=w209) -> (reference out=w207:refnum<vi>, error out=w208:errorcluster, "FP.State"=w206:T3)
                    n70 = case shown="\"Closed\"" w206 {
                      tunnel: [w214 w217] -> w211
                      tunnel: w208 -> [w213 w217]
                      tunnel: w207 -> [w212 _]
                      frame "Closed" {
                        n71 = invoke class="VI" method="FP.Open"(reference=w212, error in=w213, "Activate"=TRUE, "State"=T3."Standard") -> (error out=w214:errorcluster)  [unwired: 1 in, 4 out]
                      }
                      frame Default {
                      }
                    }
                  }
                  frame "Close" {
                    n72 = property class="VI"(reference=w220, error in=w222) -> (reference out=w219:refnum<vi>, error out=w221:errorcluster, "FP.State"=w218:T3)
                    n73 = case shown="Default" w218 {
                      tunnel: [w224 w227] -> w223
                      tunnel: w221 -> [w224 w226]
                      tunnel: w219 -> [_ w225]
                      frame "Invalid", "Closed" {
                      }
                      frame Default {
                        n74 = invoke class="VI" method="FP.Close"(reference=w225, error in=w226) -> (error out=w227:errorcluster)  [unwired: 1 in, 2 out]
                      }
                    }
                  }
                }
              }
              frame condition #1 {
              }
            }
            n75 = call <vilib>:"Add State(s) to Queue__jki_lib_state_machine.vi"("State(s) in (\"\")"=w201) -> ("States Out"=w200:string)  [unwired: 14 in]
          }
          frame "---------- Macro ----------" {
            # "Do not put any code in this frame.\n(It is a separator no-op. You can make a copy of this frame to create a new Macro frame)"
            n76 = call <vilib>:"Add State(s) to Queue__jki_lib_state_machine.vi"("State(s) in (\"\")"=w233) -> ("States Out"=w232:string)  [unwired: 14 in]
          }
          frame "Macro: Initialize" {
            w238 = "//UI: Initialize\n//UI: Front Panel State >> Open"  # //UI: Initialize //UI: Front Panel State >> Open
            w234 = "Process: Sync"
            # "Initialization Macro\n(This is called once, when the VI starts)"
            n77 = control-ref of="This VI"() -> (w236:refnum<vi>)
            n78 = property class="VI"(reference=w236) -> ("Exec.State"=w235:T4)  [unwired: 1 in, 2 out]
            n79 = Equal?(x=w235, y=T4."Run top level") -> (x = y?=w241:bool)
            n80 = Select(t=w234, s=w241, f="") -> ()  [unwired: 1 out]
            n81 = call <vilib>:"Add State(s) to Queue__jki_lib_state_machine.vi"("State(s) in Front (\"\")"="Data: Initialize\nInitialize Core Data\nEvents: Register", "State(s) in (\"\")"=w234, "State(s) at Back (\"\")"=w238) -> ("States Out"=w237:string)  [unwired: 12 in]
            n82 = call <vilib>:"Add State(s) to Queue__jki_lib_state_machine.vi"("State(s) in Front (\"\")"=w237, "State(s) in (\"\")"=w247) -> ("States Out"=w246:string)  [unwired: 13 in]
          }
          frame "Macro: Experiments" {
            # "Experimental Macros:\n- IV\n- Lockin_time\n- Lockin_Vsg\n- Lockin_sweep\n- Lockin_AIWFM_time\n- Sweep_AIWFM_time \n- Lockin?\n- THz_TimeDelay"
            # "Macro: Experiments\n(Placeholder for experiment macros)"
            n83 = call <vilib>:"Add State(s) to Queue__jki_lib_state_machine.vi"("State(s) in (\"\")"=w252) -> ("States Out"=w251:string)  [unwired: 14 in]
          }
          frame "Macro: Exit" {
            # "Exit Macro\n(This is called once, when the VI exits)"
            n84 = Unbundle By Name(w257) -> ("Core.Close Panel on Exit?"=w263:bool)
            n85 = Select(t="UI: Front Panel State >> Close", s=w263, f="") -> (s? t:f=w260:string)
            n86 = call <vilib>:"Add State(s) to Queue__jki_lib_state_machine.vi"("State(s) in Front (\"\")"="Data: Cleanup\nEvents: Unregister", "State(s) in (\"\")"="Process: Sync", "State(s) at Back (\"\")"="Exit") -> ("States Out"=w254:string)  [unwired: 12 in]
            n87 = call <vilib>:"Add State(s) to Queue__jki_lib_state_machine.vi"("State(s) in (\"\")"=w260, "State(s) at Back (\"\")"=w254) -> ("States Out"=w259:string)  [unwired: 13 in]
            n88 = call <vilib>:"Add State(s) to Queue__jki_lib_state_machine.vi"("State(s) in Front (\"\")"=w259, "State(s) in (\"\")"=w266) -> ("States Out"=w265:string)  [unwired: 13 in]
          }
          frame "---------- Process ----------" {
            # "Template Separator\n(You can make a copy of, or modify, this frame)"
            n89 = call <vilib>:"Add State(s) to Queue__jki_lib_state_machine.vi"("State(s) in (\"\")"=w271) -> ("States Out"=w270:string)  [unwired: 14 in]
          }
          frame "Process: Sync" {
            n90 = Unbundle By Name(w279) -> ("Self Reference"=w275:refnum<class "Transport.lvclass">)
            n91 = call <vilib>:"WaitOnProcessSync.vi"("error in (no error)"=w274, "SMO"=w275) -> ("error out"=w273:errorcluster, "Don't run?"=w278:bool)  [unwired: 7 in, 1 out]
            n92 = Select(t="Data: Cleanup\nEvents: Unregister\nExit", s=w278, f="") -> (s? t:f=w272:string)
            n93 = call <vilib>:"Add State(s) to Queue__jki_lib_state_machine.vi"("State(s) in Front (\"\")"=w272, "State(s) in (\"\")"=w282) -> ("States Out"=w281:string)  [unwired: 13 in]
          }
          frame "---------- Events ----------" {
            # "Template Separator\n(You can make a copy of, or modify, this frame)"
            n94 = call <vilib>:"Add State(s) to Queue__jki_lib_state_machine.vi"("State(s) in (\"\")"=w287) -> ("States Out"=w286:string)  [unwired: 14 in]
          }
          frame "Events: Register" {
            # "Expand to add\nmore events"
            n95 = Unbundle By Name(w297) -> ("Self Reference"=w290:refnum<class "Transport.lvclass">)
            n96 = call <vilib>:"GetProtectedEvents.vi"("SMO"=w290) -> ("error out"=w291:errorcluster, "SMO Protected Events"=w295:T10)  [unwired: 8 in, 1 out]
            n97 = call "Transport.GetPrivateEvents.vi"("Transport"=w290) -> ("error out"=w288:errorcluster, "Private Events"=w289:T11)  [unwired: 8 in, 1 out]
            n98 = register-events(w295, w289) -> (reference out=w296:refnum<event-registration>, error out=w292:errorcluster)  [unwired: 2 in]
            n99 = Merge Errors(w288, w294, w292, w291) -> (w293:errorcluster)
            n100 = call <vilib>:"Add State(s) to Queue__jki_lib_state_machine.vi"("State(s) in (\"\")"=w299) -> ("States Out"=w298:string)  [unwired: 14 in]
          }
          frame "Events: Unregister" {
            n101 = Unregister For Events(event registration refnum=w302, error in=w301) -> (error out=w300:errorcluster)
            n102 = call <vilib>:"Clear Errors.vi"("error in (no error)"=w300) -> ()  [unwired: 5 in, 2 out]
            n103 = call <vilib>:"Add State(s) to Queue__jki_lib_state_machine.vi"("State(s) in (\"\")"=w305) -> ("States Out"=w304:string)  [unwired: 14 in]
          }
          frame "---------- Set ----------" {
            n104 = call <vilib>:"Add State(s) to Queue__jki_lib_state_machine.vi"("State(s) in (\"\")"=w310) -> ("States Out"=w309:string)  [unwired: 14 in]
          }
          frame "Set: Wait" {
            # "#todo\nadd comments"
            n105 = Unbundle By Name(w321) -> ("wait"=w318:bool)
            n106 = call "Wait SubVI.vi"("time (ms)"=w314, "waiting"=w318) -> ("keep waiting"=w317:bool)  [unwired: 8 in, 1 out]
            n107 = call <vilib>:"Build State String with Arguments__JKI_lib_State_Machine.vi"("Arguments (\"\")"=w314, "State"=w313) -> ("State with Arguments"=w312:string)  [unwired: 4 in]
            n108 = call <vilib>:"Add State(s) to Queue__jki_lib_state_machine.vi"("State(s) in Front (\"\")"="Idle" ("format string"), "State(s) at Back (\"\")"=w312) -> ("States Out"=w311:string)  [unwired: 13 in]
            n109 = Bundle By Name(cluster=w321, "wait"=w317) -> (w320:T8)
            n110 = Select(t=w311, s=w317, f="") -> (s? t:f=w319:string)
            n111 = call <vilib>:"Add State(s) to Queue__jki_lib_state_machine.vi"("State(s) in Front (\"\")"=w319, "State(s) in (\"\")"=w325) -> ("States Out"=w324:string)  [unwired: 13 in]
          }
          frame "Set: Temperature" {
            # "#todo\nconvert string parm\nto data\n....JSON RPC?"
            n112 = Unbundle By Name(w331) -> ("Instruments.Temperature"=w328:refnum<class "Instrument.Cryostat.lvclass">)
            n113 = flat-sequence {
              tunnel: w326 -> [_]
              tunnel: [0.0 ("Target Field (T)")] -> w330
              tunnel: [0.0 ("Target Rate (T/min)")] -> w329
              frame #0 {
              }
            }
            n114 = call-dynamic "Set Temperature.vi"("error in (no error)"=w327, "Rate (K/min)"=w329, "Temperature (K)"=w330, "Instrument.Cryostat in"=w328) -> ("error out"=w332:errorcluster)  [unwired: 6 in, 1 out]
            n115 = call <vilib>:"Add State(s) to Queue__jki_lib_state_machine.vi"("State(s) in (\"\")"=w335) -> ("States Out"=w334:string)  [unwired: 14 in]
          }
          frame "Set: Magnet" {
            n116 = Unbundle By Name(w345) -> ("Instruments.Magnet"=w339:refnum<class "Instrument.Cryostat.lvclass">)
            n117 = flat-sequence {
              tunnel: w344 -> [_]
              tunnel: [0.0 ("Target Field (T)")] -> w343
              tunnel: [0.0 ("Target Rate (T/min)")] -> w342
              tunnel: [Magnet_Axis--Enum."Z" ("Axis")] -> w341
              tunnel: [Magnet_Mode--Enum."Persistent" ("Mode")] -> w340
              frame #0 {
              }
            }
            n118 = call-dynamic "Set Magnet Field.vi"("Mode"=w340, "Axis"=w341, "error in (no error)"=w338, "Target Rate (T/min)"=w342, "Target Field (T)"=w343, "Instrument.Cryostat in"=w339) -> ("error out"=w346:errorcluster)  [unwired: 4 in, 1 out]
            n119 = call <vilib>:"Add State(s) to Queue__jki_lib_state_machine.vi"("State(s) in (\"\")"=w349) -> ("States Out"=w348:string)  [unwired: 14 in]
          }
          frame "Set: Strain" {
            n120 = Unbundle By Name(w359) -> ("Instruments.Strain Cell"=w355:refnum<class "Instrument.Strain.lvclass">)
            n121 = flat-sequence {
              tunnel: w358 -> [_]
              tunnel: [0.0 ("Target Field (T)")] -> w357
              tunnel: [0.0 ("Target Rate (T/min)")] -> w356
              frame #0 {
              }
            }
            n122 = call-dynamic "Set Strain.vi"("error in (no error)"=w354, "Slew (V/s)"=w356, "Strain (V)"=w357, "Instrument.Strain in"=w355) -> ("error out"=w360:errorcluster)  [unwired: 6 in, 1 out]
            n123 = call <vilib>:"Add State(s) to Queue__jki_lib_state_machine.vi"("State(s) in (\"\")"=w363) -> ("States Out"=w362:string)  [unwired: 14 in]
          }
          frame "Set: Delay" {
            n124 = Unbundle By Name(w371) -> ("Instruments.Optical Delay Line"=w367:refnum<class "Instrument.OpticalDelayLine.lvclass">)
            n125 = flat-sequence {
              tunnel: w370 -> [_]
              tunnel: [0.0 ("Target Field (T)")] -> w369
              tunnel: [0.0 ("Target Rate (T/min)")] -> w368
              frame #0 {
              }
            }
            n126 = call-dynamic "Set Delay.vi"("error in (no error)"=w366, "Rate (ps/s)"=w368, "Delay (ps)"=w369, "Instrument.Delay in"=w367) -> ("error out"=w372:errorcluster)  [unwired: 6 in, 1 out]
            n127 = call <vilib>:"Add State(s) to Queue__jki_lib_state_machine.vi"("State(s) in (\"\")"=w375) -> ("States Out"=w374:string)  [unwired: 14 in]
          }
          frame "Set: Lockin Channel Offset" {
            n128 = Unbundle By Name(w383) -> ("Instruments.Lockin"=w379:refnum<class "Instrument.Lockin.lvclass">)
            n129 = flat-sequence {
              tunnel: w382 -> [_]
              tunnel: [0 ("Target Field (T)")] -> w381
              tunnel: [0.0 ("Target Rate (T/min)")] -> w380
              frame #0 {
              }
            }
            n130 = call <userlib>:"setAO_DC.vi"("error in (no error)"=w378, "DC (V)"=w380, "AO Channel"=w381, "Instrument.Lockin in"=w379) -> ("error out"=w384:errorcluster)  [unwired: 6 in, 1 out]
            n131 = call <vilib>:"Add State(s) to Queue__jki_lib_state_machine.vi"("State(s) in (\"\")"=w387) -> ("States Out"=w386:string)  [unwired: 14 in]
          }
          frame "Set: Lockin Channel Amplitude" {
            n132 = Unbundle By Name(w395) -> ("Instruments.Lockin"=w391:refnum<class "Instrument.Lockin.lvclass">)
            n133 = flat-sequence {
              tunnel: w394 -> [_]
              tunnel: [0 ("Target Field (T)")] -> w393
              tunnel: [0.0 ("Target Rate (T/min)")] -> w392
              frame #0 {
              }
            }
            n134 = call <userlib>:"setAO_Amp.vi"("error in (no error)"=w390, "Amplitude (V)"=w392, "AO Channel"=w393, "Instrument.Lockin in"=w391) -> ("error out"=w396:errorcluster)  [unwired: 6 in, 1 out]
            n135 = call <vilib>:"Add State(s) to Queue__jki_lib_state_machine.vi"("State(s) in (\"\")"=w399) -> ("States Out"=w398:string)  [unwired: 14 in]
          }
          frame "Set: Lockin Channel Frequency" {
            n136 = Unbundle By Name(w407) -> ("Instruments.Lockin"=w403:refnum<class "Instrument.Lockin.lvclass">)
            n137 = flat-sequence {
              tunnel: w406 -> [_]
              tunnel: [0 ("Target Field (T)")] -> w405
              tunnel: [0.0 ("Target Rate (T/min)")] -> w404
              frame #0 {
              }
            }
            n138 = call <userlib>:"setAO_f.vi"("error in (no error)"=w402, "Frequency (Hz)"=w404, "AO Channel"=w405, "Instrument.Lockin in"=w403) -> ("error out"=w408:errorcluster)  [unwired: 6 in, 1 out]
            n139 = call <vilib>:"Add State(s) to Queue__jki_lib_state_machine.vi"("State(s) in (\"\")"=w411) -> ("States Out"=w410:string)  [unwired: 14 in]
          }
          frame "Set: Lockin Channel Phase" {
            n140 = Unbundle By Name(w419) -> ("Instruments.Lockin"=w415:refnum<class "Instrument.Lockin.lvclass">)
            n141 = flat-sequence {
              tunnel: w418 -> [_]
              tunnel: [0 ("Target Field (T)")] -> w417
              tunnel: [0.0 ("Target Rate (T/min)")] -> w416
              frame #0 {
              }
            }
            n142 = call <userlib>:"setAO_phi.vi"("error in (no error)"=w414, "Phase (°)"=w416, "AO Channel"=w417, "Instrument.Lockin in"=w415) -> ("error out"=w420:errorcluster)  [unwired: 6 in, 1 out]
            n143 = call <vilib>:"Add State(s) to Queue__jki_lib_state_machine.vi"("State(s) in (\"\")"=w423) -> ("States Out"=w422:string)  [unwired: 14 in]
          }
          frame "Set: Lockin Channel Function" {
            n144 = Unbundle By Name(w431) -> ("Instruments.Lockin"=w427:refnum<class "Instrument.Lockin.lvclass">)
            n145 = flat-sequence {
              tunnel: w430 -> [_]
              tunnel: [0 ("Target Field (T)")] -> w429
              tunnel: [0.0 ("Target Rate (T/min)")] -> w428
              frame #0 {
              }
            }
            n146 = call <userlib>:"setAO_function.vi"("error in (no error)"=w426, "Function"=w428, "AO Channel"=w429, "Instrument.Lockin in"=w427) -> ("error out"=w432:errorcluster)  [unwired: 6 in, 1 out]
            n147 = call <vilib>:"Add State(s) to Queue__jki_lib_state_machine.vi"("State(s) in (\"\")"=w435) -> ("States Out"=w434:string)  [unwired: 14 in]
          }
          frame "---------- Lockin Sweep ----------" {
            n148 = call <vilib>:"Add State(s) to Queue__jki_lib_state_machine.vi"("State(s) in (\"\")"=w442) -> ("States Out"=w441:string)  [unwired: 14 in]
          }
          frame "Lockin Sweep: Configure" {
            n149 = Unbundle By Name(w446) -> ("Instruments.Lockin"=w445:refnum<class "Instrument.Lockin.lvclass">)
            n150 = call <userlib>:"setSweepConfiguration.vi"("error in (no error)"=w444, "Instrument.Lockin in"=w445) -> ("error out"=w443:errorcluster)  [unwired: 8 in, 1 out]
            n151 = call <vilib>:"Add State(s) to Queue__jki_lib_state_machine.vi"("State(s) in (\"\")"=w449) -> ("States Out"=w448:string)  [unwired: 14 in]
          }
          frame "Lockin Sweep: Start" {
            n152 = Unbundle By Name(w455) -> ("Instruments.Lockin"=w454:refnum<class "Instrument.Lockin.lvclass">)
            n153 = call <userlib>:"startSweep.vi"("error in (no error)"=w453, "Instrument.Lockin in"=w454) -> ("error out"=w451:errorcluster, "Instrument.Lockin out"=w452:refnum<class "Instrument.Lockin.lvclass">)  [unwired: 8 in]
            n154 = call <userlib>:"waitStatusSweepingStarted.vi"("error in (no error)"=w451, "Instrument.Lockin in"=w452) -> ("error out"=w450:errorcluster)  [unwired: 8 in, 1 out]
            n155 = call <vilib>:"Add State(s) to Queue__jki_lib_state_machine.vi"("State(s) in (\"\")"=w458) -> ("States Out"=w457:string)  [unwired: 14 in]
          }
          frame "Lockin Sweep: Stop" {
            n156 = Unbundle By Name(w464) -> ("Instruments.Lockin"=w463:refnum<class "Instrument.Lockin.lvclass">)
            n157 = call <userlib>:"stopSweep.vi"("error in (no error)"=w462, "Instrument.Lockin in"=w463) -> ("error out"=w460:errorcluster, "Instrument.Lockin out"=w461:refnum<class "Instrument.Lockin.lvclass">)  [unwired: 8 in]
            n158 = call <userlib>:"waitStatusSweepingStopped.vi"("error in (no error)"=w460, "Instrument.Lockin in"=w461) -> ("error out"=w459:errorcluster)  [unwired: 8 in, 1 out]
            n159 = call <vilib>:"Add State(s) to Queue__jki_lib_state_machine.vi"("State(s) in (\"\")"=w467) -> ("States Out"=w466:string)  [unwired: 14 in]
          }
          frame "Lockin Sweep: Status" {
            # "#todo\ndo stuff?"
            n160 = Unbundle By Name(w472) -> ("Instruments.Lockin"=w471:refnum<class "Instrument.Lockin.lvclass">)
            n161 = call <userlib>:"getStatus.vi"("error in (no error)"=w470, "Instrument.Lockin"=w471) -> ("error out"=w469:errorcluster, "Status"=w468:T12)  [unwired: 7 in, 1 out]
            n162 = case shown="\"idle\", Default" w468 {
              frame "idle", Default {
              }
              frame "created" {
              }
              frame "started" {
              }
              frame "stopped" {
              }
              frame "sweeping" {
              }
            }
            n163 = call <vilib>:"Add State(s) to Queue__jki_lib_state_machine.vi"("State(s) in (\"\")"=w475) -> ("States Out"=w474:string)  [unwired: 14 in]
          }
          frame "---------- Get ----------" {
            n164 = call <vilib>:"Add State(s) to Queue__jki_lib_state_machine.vi"("State(s) in (\"\")"=w480) -> ("States Out"=w479:string)  [unwired: 14 in]
          }
          frame "Get: Time" {
            n165 = Get Date/Time In Seconds() -> (seconds since 1Jan1904=w481:timestamp)
            n166 = To Double Precision Float(number=w481) -> (double precision float=w483:dbl)
            n167 = Bundle By Name(cluster=w485, "value"=w483) -> (w484:T8)
            n168 = call <vilib>:"Add State(s) to Queue__jki_lib_state_machine.vi"("State(s) in (\"\")"=w488) -> ("States Out"=w487:string)  [unwired: 14 in]
          }
          frame "Get: Temperature" {
            n169 = Unbundle By Name(w491) -> ("Instruments.Temperature"=w490:refnum<class "Instrument.Cryostat.lvclass">)
            n170 = call-dynamic "Get Temperature.vi"("error in (no error)"=w489, "Instrument.Cryostat in"=w490) -> ("error out"=w493:errorcluster, "Temperature (K)"=w492:dbl)  [unwired: 5 in, 3 out]
            n171 = Bundle By Name(cluster=w491, "value"=w492) -> (w494:T8)
            n172 = call <vilib>:"Add State(s) to Queue__jki_lib_state_machine.vi"("State(s) in (\"\")"=w497) -> ("States Out"=w496:string)  [unwired: 14 in]
          }
          frame "Get: Magnet" {
            n173 = Unbundle By Name(w500) -> ("Instruments.Magnet"=w499:refnum<class "Instrument.Cryostat.lvclass">)
            n174 = call-dynamic "Get Magnet Field.vi"("error in (no error)"=w498, "Instrument.Cryostat in"=w499) -> ("error out"=w502:errorcluster, "B Field (T)"=w501:dbl)  [unwired: 5 in, 3 out]
            n175 = Bundle By Name(cluster=w500, "value"=w501) -> (w503:T8)
            n176 = call <vilib>:"Add State(s) to Queue__jki_lib_state_machine.vi"("State(s) in (\"\")"=w506) -> ("States Out"=w505:string)  [unwired: 14 in]
          }
          frame "Get: Capacitance" {
            n177 = Unbundle By Name(w509) -> ("Instruments.C Bridge"=w508:refnum<class "Instrument.CBridge.lvclass">)
            n178 = call-dynamic "Get Capacitance.vi"("error in (no error)"=w507, "Instrument.CBridge in"=w508) -> ("error out"=w511:errorcluster, "Capacitance (pF)"=w510:dbl)  [unwired: 7 in, 1 out]
            n179 = Bundle By Name(cluster=w509, "value"=w510) -> (w512:T8)
            n180 = call <vilib>:"Add State(s) to Queue__jki_lib_state_machine.vi"("State(s) in (\"\")"=w515) -> ("States Out"=w514:string)  [unwired: 14 in]
          }
          frame "Get: Strain" {
            n181 = Unbundle By Name(w518) -> ("Instruments.Strain Cell"=w517:refnum<class "Instrument.Strain.lvclass">)
            n182 = call-dynamic "Get Strain.vi"("error in (no error)"=w516, "Instrument.Strain in"=w517) -> ("error out"=w520:errorcluster, "Strain (V)"=w519:dbl)  [unwired: 7 in, 1 out]
            n183 = Bundle By Name(cluster=w518, "value"=w519) -> (w521:T8)
            n184 = call <vilib>:"Add State(s) to Queue__jki_lib_state_machine.vi"("State(s) in (\"\")"=w524) -> ("States Out"=w523:string)  [unwired: 14 in]
          }
          frame "Get: Delay" {
            n185 = Unbundle By Name(w527) -> ("Instruments.Optical Delay Line"=w526:refnum<class "Instrument.OpticalDelayLine.lvclass">)
            n186 = call-dynamic "Get Delay.vi"("error in (no error)"=w525, "Instrument.Delay in"=w526) -> ("error out"=w529:errorcluster, "Delay (ps)"=w528:dbl)  [unwired: 6 in, 2 out]
            n187 = Bundle By Name(cluster=w527, "value"=w528) -> (w530:T8)
            n188 = call <vilib>:"Add State(s) to Queue__jki_lib_state_machine.vi"("State(s) in (\"\")"=w533) -> ("States Out"=w532:string)  [unwired: 14 in]
          }
          frame "Get: Lockin AO" {
            n189 = Unbundle By Name(w536) -> ("Instruments.Lockin"=w535:refnum<class "Instrument.Lockin.lvclass">)
            n190 = call <userlib>:"getAO.vi"("error in (no error)"=w534, "Instrument.Lockin in"=w535) -> ("error out"=w538:errorcluster, "AO Waveforrm"=w537:waveform(dbl)[])  [unwired: 7 in, 1 out]
            n191 = Bundle By Name(cluster=w536, "value"=w537) -> (w539:T8)
            n192 = call <vilib>:"Add State(s) to Queue__jki_lib_state_machine.vi"("State(s) in (\"\")"=w542) -> ("States Out"=w541:string)  [unwired: 14 in]
          }
          frame "Get: Lockin AI" {
            n193 = Unbundle By Name(w545) -> ("Instruments.Lockin"=w544:refnum<class "Instrument.Lockin.lvclass">)
            n194 = call <userlib>:"getAI.vi"("error in (no error)"=w543, "Instrument.Lockin in"=w544) -> ("error out"=w547:errorcluster, "AI Waveform"=w546:waveform(dbl)[])  [unwired: 7 in, 1 out]
            n195 = Bundle By Name(cluster=w545, "value"=w546) -> (w548:T8)
            n196 = call <vilib>:"Add State(s) to Queue__jki_lib_state_machine.vi"("State(s) in (\"\")"=w551) -> ("States Out"=w550:string)  [unwired: 14 in]
          }
          frame "Get: Lockin Result" {
            n197 = Unbundle By Name(w554) -> ("Instruments.Lockin"=w553:refnum<class "Instrument.Lockin.lvclass">)
            n198 = call <userlib>:"getResults.vi"("error in (no error)"=w552, "Instrument.Lockin in"=w553) -> ("error out"=w556:errorcluster, "Results (Dictionary)"=w555:cluster{"key":string, "value":dbl}[])  [unwired: 6 in, 2 out]
            n199 = Bundle By Name(cluster=w554, "value"=w555) -> (w557:T8)
            n200 = call <vilib>:"Add State(s) to Queue__jki_lib_state_machine.vi"("State(s) in (\"\")"=w560) -> ("States Out"=w559:string)  [unwired: 14 in]
          }
        }
      }
    }
    frame Error {
    }
  }
  n201 = call-parent "Process.vi"("error in"=w7, "SMO"=w6) -> ("error out"=w4:errorcluster, "SMO out"=→"Transport out":refnum<class "Transport.lvclass">)  [unwired: 8 in]
  n202 = Merge Errors(w4, w3) -> (→"error out":errorcluster)
